vi "Display_OutputVGAsignal.vi"(1 "Red":bool, 2 "Green":bool, 3 "Blue":bool, 4 "ActivePixel":T1, 6 "Blue [FPGA DO]":refnum<k21>, 7 "h_sync [FPGA DO]":refnum<k21>, 8 "Green  [FPGA DO]":refnum<k21>, 9 "v_sync [FPGA DO]":refnum<k21>, 10 "Red  [FPGA DO]":refnum<k21>) -> ()   [LabVIEW 2018]
uses:
  TypDefs/ActivePixel_Cluster.ctl
  <vilib>/rvi/eio/common/nirviEmuTemplateMethod_errors.vi
  <vilib>/eio/EIONode/EIONode.xnode
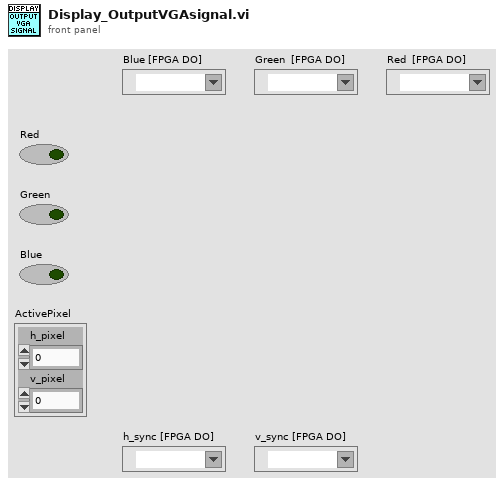
[diagram p1: front panel]
types:
  T1 = typedef "ActivePixel_Cluster.ctl" = cluster{"h_pixel":i16, "v_pixel":i16}
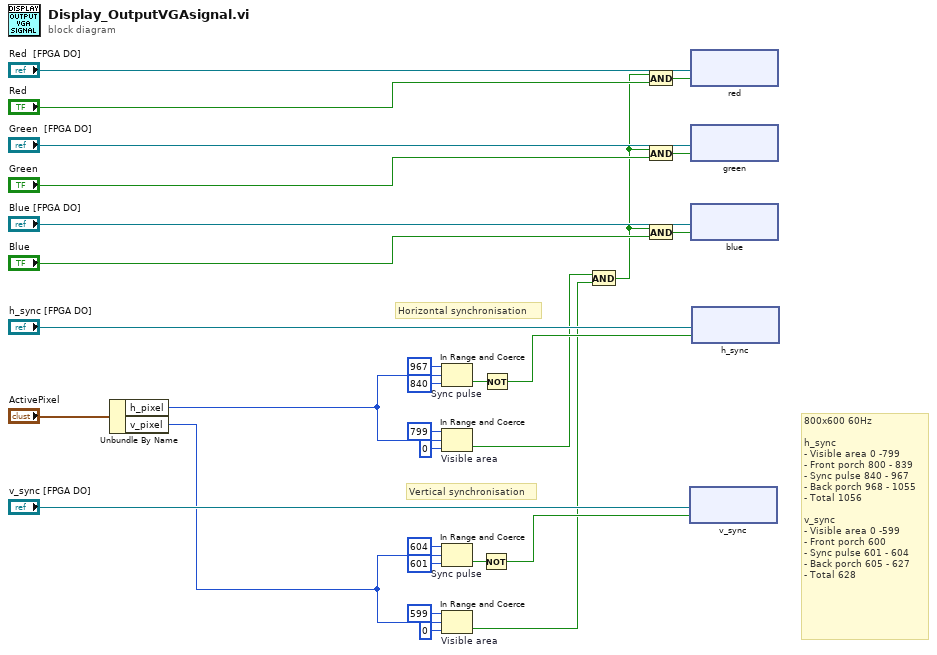
[diagram p0: block diagram]
diagram:
  # "Vertical synchronisation"
  # "Horizontal synchronisation"
  # "800x600 60Hz\n\nh_sync\n- Visible area 0 -799\n- Front porch 800 - 839\n- Sync pulse 840 - 967\n- Back porch 968 - 1055\n- Total 1056\n\nv_sync\n- Visible area 0 -599\n- Front porch 600\n- Sync pulse 601 - 604\n- Back porch 605 - 627\n- Total 628"
  n1 = Unbundle By Name("ActivePixel") -> ("h_pixel"=w5:i16, "v_pixel"=w4:i16)
  n2 = In Range and Coerce "Sync pulse"(upper limit=i16 967, x=w5, lower limit=i16 840) -> (In Range?=w27:bool)  [unwired: 1 out]
  n3 = In Range and Coerce "Visible area"(upper limit=i16 799, x=w5, lower limit=i16 0) -> (In Range?=w2:bool)  [unwired: 1 out]
  n4 = In Range and Coerce "Sync pulse"(upper limit=i16 604, x=w4, lower limit=i16 601) -> (In Range?=w12:bool)  [unwired: 1 out]
  n5 = In Range and Coerce "Visible area"(upper limit=i16 599, x=w4, lower limit=i16 0) -> (In Range?=w1:bool)  [unwired: 1 out]
  n6 = Not(x=w12) -> (.not. x?=w7:bool)
  n7 = Not(x=w27) -> (.not. x?=w23:bool)
  n8 = And(x=w2, y=w1) -> (x .and. y?=w3:bool)
  n9 = And(x=w3, y="Red") -> (x .and. y?=w18:bool)
  n10 = And(x=w3, y="Green") -> (x .and. y?=w17:bool)
  n11 = And(x=w3, y="Blue") -> (x .and. y?=w16:bool)
  n12 = xnode "v_sync"("I/O Item"=w7, "FPGA I/O In"="v_sync [FPGA DO]") -> ()  [unwired: 1 out]
  n13 = xnode "red"("I/O Item"=w18, "FPGA I/O In"="Red  [FPGA DO]") -> ()  [unwired: 1 out]
  n14 = xnode "green"("I/O Item"=w17, "FPGA I/O In"="Green  [FPGA DO]") -> ()  [unwired: 1 out]
  n15 = xnode "blue"("I/O Item"=w16, "FPGA I/O In"="Blue [FPGA DO]") -> ()  [unwired: 1 out]
  n16 = xnode "h_sync"("I/O Item"=w23, "FPGA I/O In"="h_sync [FPGA DO]") -> ()  [unwired: 1 out]
